vi "Send Synchronous Reply.vi"(8 "Return Error":errorcluster, 10 "Data (Optional)":variant, 11 "SynchronousMsg":refnum<class "SynchronousMsg.lvclass">) -> (0 "error out":errorcluster)   [LabVIEW 2015, in "AbstractMessages.lvlib" / "SynchronousMsg.lvclass"]
doc: "<License>\nCopyright © 2017 Composed Systems, LLC | All rights reserved\nwww.composed.io\n\nAuthor: Ethan Stern <ethan.stern@composed.io>\n\nThis software is provided \"AS IS\" WITHOUT WARRANTIES, either express or implied, AND IS FOR EDUCATIONAL PURPOSES ONLY.\n</License>"
uses:
  SynchronousMsg.lvclass
  SynchronousMsg.lvclass/SynchronousMsg.ctl
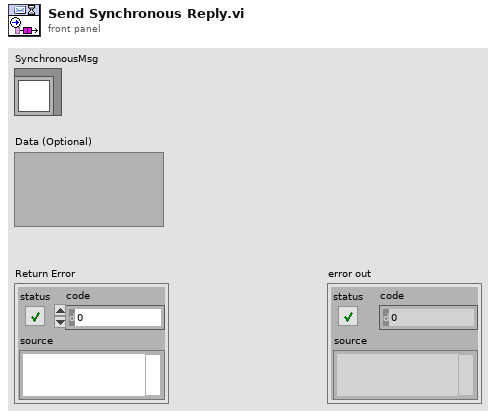
[diagram p1: front panel]
types:
  T1 = cluster{"Data (Optional)":variant, "Return Error":errorcluster}
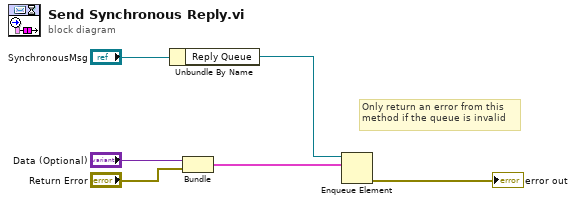
[diagram p0: block diagram]
diagram:
  # "Only return an error from this\nmethod if the queue is invalid"
  n1 = Unbundle By Name("SynchronousMsg") -> ("Reply Queue"=w5:refnum<queue>)
  n2 = Bundle("Data (Optional)"="Data (Optional)", "Return Error"="Return Error") -> (w2:T1)  [unwired: 1 in]
  n3 = Enqueue Element(queue=w5, element=w2) -> (error out=→"error out":errorcluster)  [unwired: 2 in, 2 out]
